vi "IsOverloaded.vi"(8 "Error In":errorcluster, 11 "Kiethley 2602 In":refnum<visa-resource-name>) -> (0 "Error Out":errorcluster, 2 "Overloaded?":bool, 3 "Keithley 2602 Out":refnum<visa-resource-name>)   [LabVIEW 2012, in "Keithley-2602.lvlib"]
uses:
  Keithley-2602.lvlib
  Controls/Register.ctl
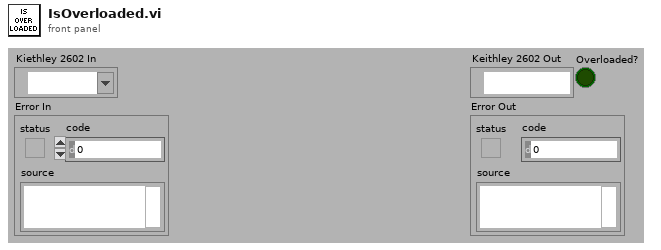
[diagram p1: front panel]
types:
  T1 = typedef "Keithley-2602.lvlib/Register.ctl" = enum16{"Condition", "Event", "Enable", "Positive Transition", "Negative Transition"}
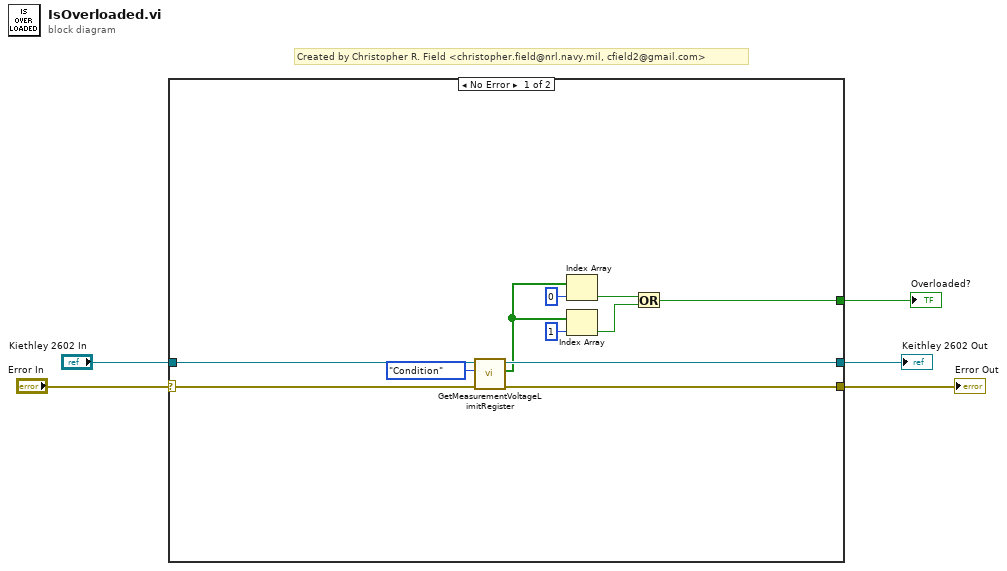
[diagram p0: block diagram]
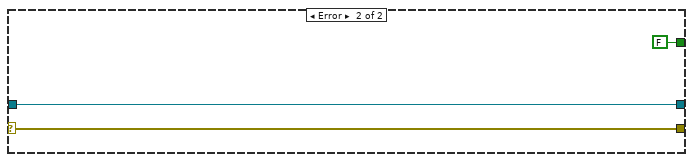
[diagram p2: hidden frame]
diagram:
  # "Created by Christopher R. Field <christopher.field@nrl.navy.mil, cfield2@gmail.com>"
  n1 = case shown="No Error" "Error In" {
    selector: "Error In" -> [w7 w19]
    tunnel: "Kiethley 2602 In" -> [w16 w18]
    tunnel: [w15 w18] -> w4
    tunnel: [w14 w19] -> w3
    tunnel: [w8 FALSE] -> w2
    frame No Error {
      n2 = call "GetMeasurementVoltageLimitRegister.vi"("Error In"=w7, "Register"=Register."Condition", "Kiethley 2602 In"=w16) -> ("Error Out"=w14:errorcluster, "Measurement Voltage Limit Register"=w13:bool[], "Keithley 2602 Out"=w15:refnum<visa-resource-name>)  [unwired: 6 in]
      n3 = Index Array(array=w13, index=0) -> (element=w10:bool)
      n4 = Index Array(array=w13, index=1) -> (element=w9:bool)
      n5 = Or(x=w10, y=w9) -> (x .or. y?=w8:bool)
    }
    frame Error {
    }
  }
  "Keithley 2602 Out" <- w4
  "Error Out" <- w3
  "Overloaded?" <- w2
